vi "Lookup Session Value.vi"(8 "error in (no error)":errorcluster, 10 "Name":string, 11 "Processing in":refnum<class "Processing.lvclass">) -> (0 "error out":errorcluster, 1 "Not Found?":bool, 2 "Value":string, 3 "Processing out":refnum<class "Processing.lvclass">)   [LabVIEW 2020, in "HTTP Server.lvlib" / "Processing.lvclass"]
uses:
  Processing.lvclass
  Session/Session.lvclass
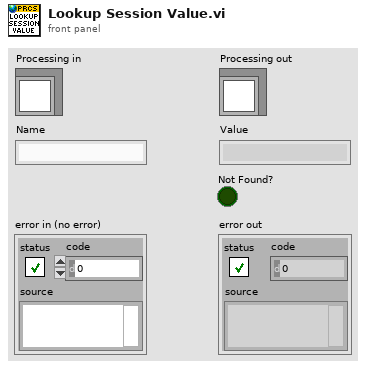
[diagram p1: front panel]
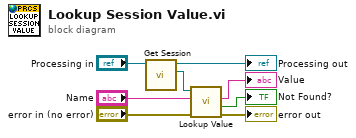
[diagram p0: block diagram]
diagram:
  n1 = call "Get Session.vi"("Processing in"="Processing in") -> ("Session"=w7:refnum<class "Session.lvclass">, "Processing out"=→"Processing out":refnum<class "Processing.lvclass">)  [unwired: 9 in]
  n2 = call "Lookup Value.vi"("error in (no error)"="error in (no error)", "Name"="Name", "Session in"=w7) -> ("error out"=→"error out":errorcluster, "Not Found?"=→"Not Found?":bool, "Value"=→"Value":string)  [unwired: 5 in, 1 out]
